vi "HFRR ADV v011 new software.vi"() -> ()   [LabVIEW 2025] (continued)
            n4020 = Unbundle(w5344) -> ("status"=w5343:bool)  [unwired: 2 out]
            n4021 = case shown="True" w5343 {
              selector: w5343 -> [_ w5360]
              frame False {
              }
              frame True {
                n4022 = local write "TK4 status"(w5360) -> ()
              }
            }
          }
        }
        n4023 = local read "Quit"() -> (w5264:bool)
      }
      n4024 = VISA Close(VISA resource name=w5260, error in (no error)=w5261) -> (error out=w5259:errorcluster)
      n4025 = call <vilib>:"Clear Errors.vi"("error in (no error)"=w5259) -> ()  [unwired: 5 in, 2 out]
    }
    frame Enabled {
    }
  }
